vi "Sample Report (Excel).vi"() -> ()   [LabVIEW 2020]
doc: "The purpose of this example is to show how to use the high-level Excel specific VIs to generate a test report."
uses:
  <vilib>/addons/_office/excel.llb/Excel Easy Table (str).vi
  <vilib>/Utility/NIReport.llb/NI_report.lvclass
  <vilib>/addons/_office/NI_ReportGenerationToolkit.lvlib
  <vilib>/Utility/NIReport.llb/Excel/NI_Excel.lvclass
panel:
  in  "Text":string="Description: the purpose of this example is to show how to use the high-level Excel specific VIs to generate a test report.\n\n\n\n\n\n\n"
  in  "Table":string[][](table)=[["1", "1.5", "5.6", "5.6", "7.9", "4.6"], ["2", "2.5", "7.6", "6.5", "7.2", "7.5"], ["3", "6.8", "9.1", "4.2", "6.2", "6.1"], ["4", "6.7", "7.1", "7.2", "1.0", "8.3"], ["5", "6.4", "4.3", "9.2", "5.8", "4.2"], ["6", "8.6", "8.2", "4.3", "8.6", "4.5"]]
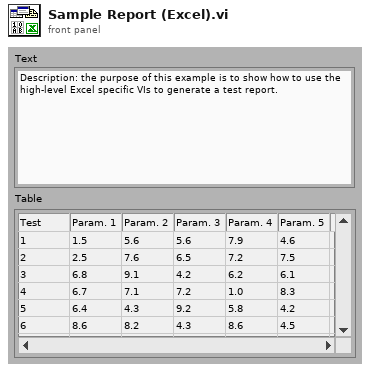
[diagram p1: front panel]
types:
  T1 = enum16{"Standard Report", "HTML", "Word", "Excel"}
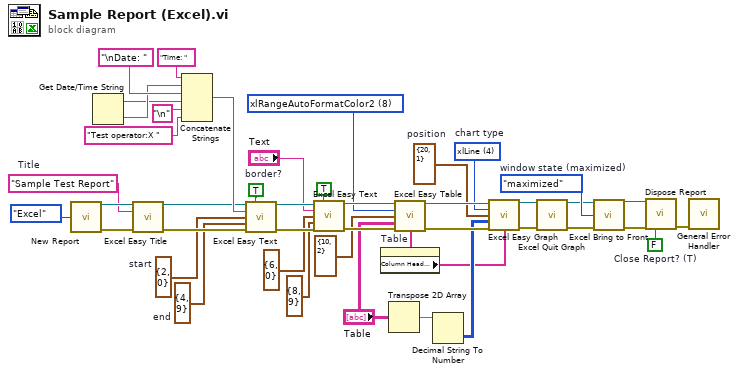
[diagram p0: block diagram]
diagram:
  w28 = "Sample Test Report"  # Title
  w1 = FALSE  # Close Report? (T)
  w9 = enum16{"maximized", "minimized", "normal"}."maximized"  # window state (maximized)
  w16 = 8 items=["xlRangeAutoFormat3DEffects1"=13, "xlRangeAutoFormat3DEffects2"=14, "xlRangeAutoFormatAccounting1"=4, "xlRangeAutoFormatAccounting2"=5, "xlRangeAutoFormatAccounting3"=6, "xlRangeAutoFormatAccounting4"=17, "xlRangeAutoFormatClassic1"=1, "xlRangeAutoFormatClassic2"=2, "xlRangeAutoFormatClassic3"=3, "xlRangeAutoFormatColor1"=7, "xlRangeAutoFormatColor2"=8, "xlRangeAutoFormatColor3"=9, "xlRangeAutoFormatList1"=10, "xlRangeAutoFormatList2"=11, "xlRangeAutoFormatList3"=12, "xlRangeAutoFormatLocalFormat1"=15, "xlRangeAutoFormatLocalFormat2"=16, "xlRangeAutoFormatLocalFormat3"=19, "xlRangeAutoFormatLocalFormat4"=20, "xlRangeAutoFormatReport1"=21, "xlRangeAutoFormatReport2"=22, "xlRangeAutoFormatReport3"=23, "xlRangeAutoFormatReport4"=24, "xlRangeAutoFormatReport5"=25, "xlRangeAutoFormatReport6"=26, "xlRangeAutoFormatReport7"=27, "xlRangeAutoFormatReport8"=28, "xlRangeAutoFormatReport9"=29, "xlRangeAutoFormatReport10"=30, "xlRangeAutoFormatClassicPivotTable"=31, "xlRangeAutoFormatTable1"=32, "xlRangeAutoFormatTable2"=33, "xlRangeAutoFormatTable3"=34, "xlRangeAutoFormatTable4"=35, "xlRangeAutoFormatTable5"=36, "xlRangeAutoFormatTable6"=37, "xlRangeAutoFormatTable7"=38, "xlRangeAutoFormatTable8"=39, "xlRangeAutoFormatTable9"=40, "xlRangeAutoFormatTable10"=41, "xlRangeAutoFormatPTNone"=42, "xlRangeAutoFormatNone"=-4142, "xlRangeAutoFormatSimple"=-4154] ("auto format")
  w15 = cluster{"row":i32, "column":i32} {"row"=20, "column"=1}  # position
  w11 = TRUE  # border?
  w21 = cluster{"row":i32, "column":i32} {"row"=4, "column"=9}  # end
  w22 = cluster{"row":i32, "column":i32} {"row"=2, "column"=0}  # start
  w14 = 4 items=["xlColumnClustered"=51, "xlColumnStacked"=52, "xlColumnStacked100"=53, "xl3DColumnClustered"=54, "xl3DColumnStacked"=55, "xl3DColumnStacked100"=56, "xlBarClustered"=57, "xlBarStacked"=58, "xlBarStacked100"=59, "xl3DBarClustered"=60, "xl3DBarStacked"=61, "xl3DBarStacked100"=62, "xlLineStacked"=63, "xlLineStacked100"=64, "xlLineMarkers"=65, "xlLineMarkersStacked"=66, "xlLineMarkersStacked100"=67, "xlPieOfPie"=68, "xlPieExploded"=69, "xl3DPieExploded"=70, "xlBarOfPie"=71, "xlXYScatterSmooth"=72, "xlXYScatterSmoothNoMarkers"=73, "xlXYScatterLines"=74, "xlXYScatterLinesNoMarkers"=75, "xlAreaStacked"=76, "xlAreaStacked100"=77, "xl3DAreaStacked"=78, "xl3DAreaStacked100"=79, "xlDoughnutExploded"=80, "xlRadarMarkers"=81, "xlRadarFilled"=82, "xlSurface"=83, "xlSurfaceWireframe"=84, "xlSurfaceTopView"=85, "xlSurfaceTopViewWireframe"=86, "xlBubble"=15, "xlBubble3DEffect"=87, "xlStockHLC"=88, "xlStockOHLC"=89, "xlStockVHLC"=90, "xlStockVOHLC"=91, "xlCylinderColClustered"=92, "xlCylinderColStacked"=93, "xlCylinderColStacked100"=94, "xlCylinderBarClustered"=95, "xlCylinderBarStacked"=96, "xlCylinderBarStacked100"=97, "xlCylinderCol"=98, "xlConeColClustered"=99, "xlConeColStacked"=100, "xlConeColStacked100"=101, "xlConeBarClustered"=102, "xlConeBarStacked"=103, "xlConeBarStacked100"=104, "xlConeCol"=105, "xlPyramidColClustered"=106, "xlPyramidColStacked"=107, "xlPyramidColStacked100"=108, "xlPyramidBarClustered"=109, "xlPyramidBarStacked"=110, "xlPyramidBarStacked100"=111, "xlPyramidCol"=112, "xl3DColumn"=-4100, "xlLine"=4, "xl3DLine"=-4101, "xl3DPie"=-4102, "xlPie"=5, "xlXYScatter"=-4169, "xl3DArea"=-4098, "xlArea"=1, "xlDoughnut"=-4120, "xlRadar"=-4151]  # chart type
  n1 = call <vilib>:"New Report.vi"("report type"=T1."Excel") -> ("report out"=w30:refnum<class "NI_report.lvclass">, "error out"=w32:errorcluster)  [unwired: 13 in]
  n2 = Get Date/Time String() -> (date string=w5:string, time string=w6:string)  [unwired: 3 in]
  n3 = call <vilib>:"Excel Easy Title.vi"("report in"=w30, "title"=w28, "error in (no error)"=w32) -> ("report out"=w29:refnum<class "NI_report.lvclass">, "error out"=w31:errorcluster)  [unwired: 10 in, 1 out]
  n4 = Concatenate Strings("Time: " ("Substring"), w6, "\nDate: " ("Substring"), w5, "\n" ("Substring"), "Test operator:X " ("Substring")) -> (w38:string)
  n5 = call <vilib>:"Excel Easy Text.vi"("report in"=w29, "border? (F)"=w11, "text"=w38, "start (-1, -1)"=w22, "end (-1, -1)"=w21, "error in (no error)"=w31) -> ("report out"=w36:refnum<class "NI_report.lvclass">, "error out"=w37:errorcluster)  [unwired: 5 in, 3 out]
  n6 = call <vilib>:"Excel Easy Text.vi"("report in"=w36, "border? (F)"=TRUE ("border?"), "text"="Text", "start (-1, -1)"=cluster{"row":i32, "column":i32} {"row"=6, "column"=0} ("start"), "end (-1, -1)"=cluster{"row":i32, "column":i32} {"row"=8, "column"=9} ("end"), "error in (no error)"=w37) -> ("report out"=w34:refnum<class "NI_report.lvclass">, "error out"=w35:errorcluster)  [unwired: 5 in, 3 out]
  n7 = property on="Table" class="Tbl (strict)"() -> ("Column Header Strings[]"=w18:string[])  [unwired: 2 in, 2 out]
  n8 = Transpose 2D Array(2D array="Table") -> (transposed array=w23:string[][])
  n9 = call-poly <vilib>:"Excel Easy Table.vi"("report in"=w34, "auto format (none)"=w16, "start (0, 0)"=cluster{"row":i32, "column":i32} {"row"=10, "column"=2} ("position"), "text data"="Table", "error in (no error)"=w35, "row headers"=w18) -> ("report out"=w26:refnum<class "NI_report.lvclass">, "error out"=w27:errorcluster)  [unwired: 5 in, 3 out]
  n10 = Decimal String To Number(string=w23) -> (number=w24:i32[][])  [unwired: 2 in, 1 out]
  n11 = call <vilib>:"Excel Easy Graph.vi"("report in"=w26, "graph type (col clustered)"=w14, "start (0, 0)"=w15, "data"=w24, "error in (no error)"=w27, "row headers"=w18) -> ("report out"=w12:refnum<class "NI_report.lvclass">, "error out"=w13:errorcluster)  [unwired: 8 in]
  n12 = call <vilib>:"Excel Quit Graph.vi"("report in"=w12, "error in (no error)"=w13) -> ("report out"=w7:refnum<class "NI_report.lvclass">, "error out"=w8:errorcluster)  [unwired: 12 in]
  n13 = call <vilib>:"Excel Bring to Front.vi"("report in"=w7, "window state (maximized)"=w9, "error in (no error)"=w8) -> ("report out"=w3:refnum<class "NI_report.lvclass">, "error out"=w4:errorcluster)  [unwired: 11 in]
  n14 = call-dynamic "Dispose Report.vi"("report in"=w3, "error in (no error)"=w4, "close report? (T)"=w1) -> ("error out"=w2:errorcluster)  [unwired: 12 in]
  n15 = call <vilib>:"General Error Handler.vi"("error in (no error)"=w2) -> ()  [unwired: 10 in, 5 out]
